vi "Show Tree.vi"(7 "Root ID":string, 8 "Error In":errorcluster, 10 "Show IDs (False)":bool, 11 "Tree":refnum<data-value>) -> (0 "Error Out":errorcluster, 1 "Items Out":T1(array[cluster]), 3 "Tree":refnum<data-value>)   [LabVIEW 2017, in "Tree API.lvlib" / "Tree.lvclass"]
doc: "Recursively traverse down wired Tree ID and populate the Tree Control with the contents of the Tree.\n\nBecause the Tree Control requires to have only one root element, the Root ID has to be specified. This means that if you have multiple roots in your Tree you need to visualize them seperately."
uses:
  Tree.lvclass
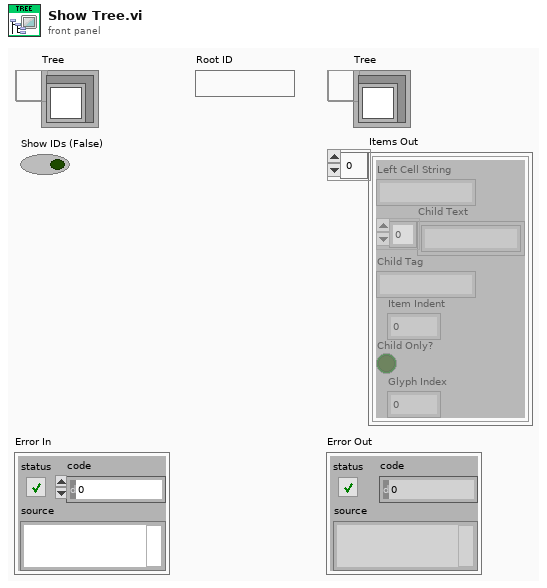
[diagram p1: front panel]
types:
  T1 = cluster{"Left Cell String":string, "Child Text":string[], "Child Tag":string, "Item Indent":i32, "Child Only?":bool, "Glyph Index":i32}[]
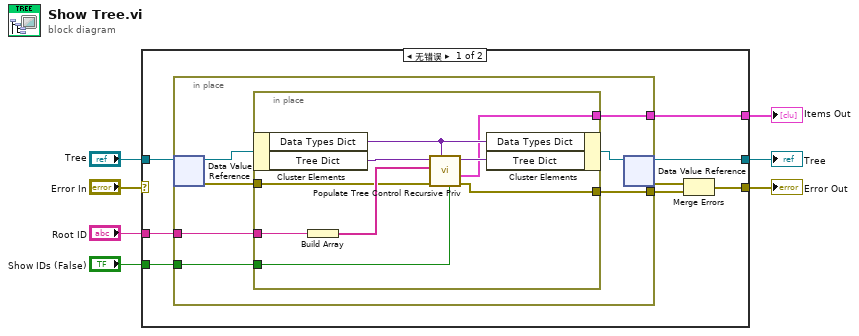
[diagram p0: block diagram]
diagram:
  n1 = case shown="无错误" "Error In" {
    selector: "Error In" -> [_ w32]
    tunnel: "Tree" -> [w15 w33]
    tunnel: [w14 w33] -> w6
    tunnel: [w8 w32] -> w4
    tunnel: "Root ID" -> [w13 _]
    tunnel: "Show IDs (False)" -> [w12 _]
    tunnel: [w11 _] -> w1
    frame No Error {
      n2 = in-place {
        in-place-border: w13 -> [w20]
        in-place-border: w12 -> [w18]
        in-place-border: [w17] -> w11
        in-place-border: [w16] -> w9
        n3 = in-place-dvr #1(w15) -> (w22:refnum<class "Tree.lvclass">, w19:errorcluster)
        n4 = in-place {
          in-place-border: w20 -> [w29]
          in-place-border: w19 -> [w25]
          in-place-border: w18 -> [w27]
          in-place-border: [w24] -> w17
          in-place-border: [w23] -> w16
          n5 = in-place-cluster #2(w22) -> ("Data Types Dict"=w26:variant, "Tree Dict"=w31:variant)
          n6 = Build Array(w29) -> (w28:string[])
          n7 = call "Populate Tree Control Recursive Priv.vi"("Show IDs (True)"=w27, "Data Types Dict"=w26, "error in"=w25, "Child IDs"=w28, "Tree Dictionary In"=w31) -> ("error out"=w23:errorcluster, "Items Out"=w24:T1, "Tree Dictionary Out"=w30:variant)  [unwired: 4 in]
          n8 = in-place-cluster #2("Data Types Dict"=w26, "Tree Dict"=w30) -> (w21:refnum<class "Tree.lvclass">)
        }
        n9 = in-place-dvr #1(w21) -> (w14:refnum<data-value>, w10:errorcluster)
      }
      n10 = Merge Errors(w10, w9) -> (w8:errorcluster)
    }
    frame Error {
    }
  }
  "Tree" <- w6
  "Error Out" <- w4
  "Items Out" <- w1
